vi "Nearest Neighbors 2D Double.vi"() -> ()   [LabVIEW 2020]
uses:
  <vilib>/numeric/Random Number (Range) DBL.vi
  Classes/KD Tree Double/KD Tree Double.lvclass
  E:/Labview/LV 2020/Libs/flann/flann/Classes/KD Tree/KD Tree.lvclass
  Classes/KD Tree Double/Create KD Tree Double.vi
  Classes/KD Tree Double/Find Nearest Neighbors Index Double.vi
  Classes/KD Tree/KD Tree.lvclass
panel:
  out "XY Graph":cluster{cluster{"number":dbl, "number":dbl}[]}[](graph)
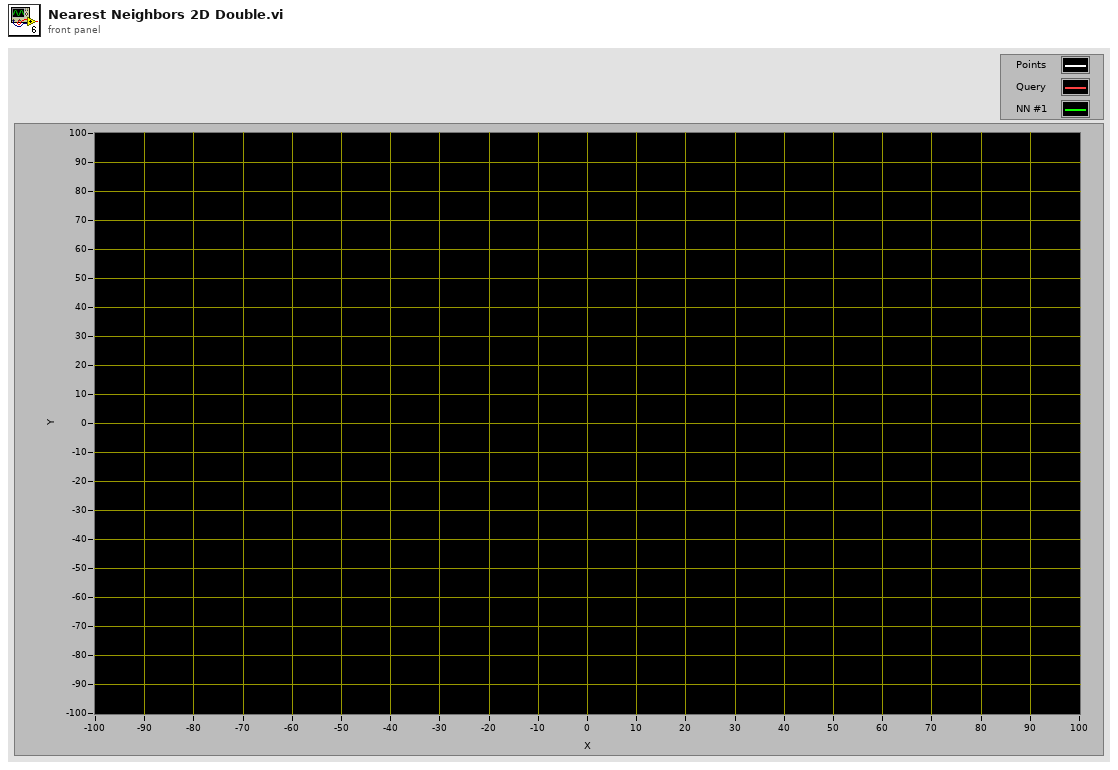
[diagram p1: front panel]
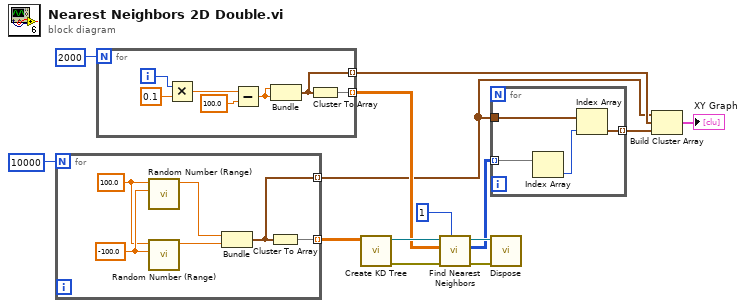
[diagram p0: block diagram]
diagram:
  n1 = for {
    N: 10000 -> [_]
    tunnel: [w20] -> w3 mode=indexing
    tunnel: [w19] -> w13 mode=indexing
    w15 = 100.0 ("lower bound (0)")
    w16 = -100.0 ("lower bound (0)")
    n2 = call-poly <vilib>:"Random Number (Range).vi"("lower bound (0)"=w16, "upper bound (100)"=w15) -> ("number"=w17:dbl)  [unwired: 9 in]
    n3 = call-poly <vilib>:"Random Number (Range).vi"("lower bound (0)"=w16, "upper bound (100)"=w15) -> ("number"=w18:dbl)  [unwired: 9 in]
    n4 = Bundle("number"=w17, "number"=w18) -> (w20:cluster{"number":dbl, "number":dbl})  [unwired: 1 in]
    n5 = Cluster To Array(cluster=w20) -> (array=w19:dbl[])
  }
  n6 = for {
    N: 2000 -> [_]
    tunnel: [w22] -> w7 mode=indexing
    tunnel: [w27] -> w5 mode=indexing
    i -> [w26]
    n7 = Multiply(x=w26, y=0.1) -> (x*y=w24:dbl)
    n8 = Subtract(x=w24, y=100.0) -> (x-y=w21:dbl)
    n9 = Bundle(w21, w21) -> (w22:cluster{dbl, dbl})  [unwired: 1 in]
    n10 = Cluster To Array(cluster=w22) -> (array=w27:dbl[])
  }
  n11 = call-poly "Create KD Tree.vi"("Points (Row-Vectors)"=w13) -> ("error out"=w11:errorcluster, "KD Tree Double out"=w12:refnum<class "KD Tree Double.lvclass">)  [unwired: 9 in]
  n12 = call-poly "Find Nearest Neighbors.vi"("#Neighbors"=1, "error in (no error)"=w11, "Points"=w5, "KD Tree Double in"=w12) -> ("error out"=w9:errorcluster, "Indices"=w2:i32[][], "KD Tree Double out"=w8:refnum<class "KD Tree Double.lvclass">)  [unwired: 4 in, 1 out]
  n13 = for {
    tunnel: w3 -> [w31]
    tunnel: w2 -> [w30] mode=indexing
    tunnel: [w28] -> w1 mode=indexing
    n14 = Index Array(array=w30) -> (element=w29:i32)  [unwired: 1 in]
    n15 = Index Array(array=w31, index=w29) -> (element=w28:cluster{"number":dbl, "number":dbl})
  }
  n16 = call "Dispose.vi"("error in (no error)"=w9, "KD Tree in"=w8) -> ()  [unwired: 9 in, 1 out]
  n17 = Build Cluster Array(w3, w7, w1) -> (→"XY Graph":cluster{cluster{"number":dbl, "number":dbl}[]}[])
